vi "Process Outgoing Messages.vi"(0 "J1939 Cluster":T10, 1 "Connection Refs":T1, 5 "Timeouts":T9[](array[typedef]) {"Arb ID" format="%.0x"}, 7 "Data Ref":T7, 9 "Scale Ref":T8, 11 "error in":errorcluster, 12 "timeout in ms (-1)":i32=10) -> (4 "J1939 Cluster Out":T10, 13 "Message Errors":errorcluster, 15 "error out":errorcluster)   [LabVIEW 2015, in "J1939 Addon Engine.lvlib"]
uses:
  J1939 Addon Engine.lvlib
  Types/Setup Information Cluster.ctl
  <vilib>/xnet/xnet.llb/XNET Frame CAN.ctl
  <vilib>/xnet/xnet.llb/XNET Frame Type CAN.ctl
  Shared/J1939 Utilities/Types/CAN Outgoing Message Cluster.ctl
  J1939 Periodic Messages/SubVIs/Periodic Message Generator Cluster.ctl
  Types/Conversion Lookup Table Reference.ctl
  Types/Data Lookup Table Reference.ctl
  Types/Datatable Lookup DVR.ctl
  Types/TP List References.ctl
  Types/BAM Buffer Connections List_Ref.ctl
  Types/TP Buffer Connection Cluster.ctl
  Types/Connection Mode Generation Connection Ref.ctl
  Types/Connection Mode Generation Connection Cluster.ctl
  Types/BAM Generation Connections List_Ref.ctl
  Types/BAM Generation Connection Cluster.ctl
  Types/Address Table Reference.ctl
  Types/RQST Lookup Table Reference.ctl
  Shared/J1939 Utilities/Check Output Message Frame Type.vi
  J1939 Multi Packet Frames/BAM Generation.vi
  SubVIs/BAM Generation Connections List_Actions.vi
  SubVIs/BAM Generation Create New TP Connection.vi
  J1939 Multi Packet Frames/Connection Mode Generation.vi
  SubVIs/Connection Mode Generation Connections List_Actions.vi
  SubVIs/Connection Mode Generation Search for Connection (Local Message).vi
  SubVIs/Connection Mode Generation Create New TP Connection.vi
  Convert Signals to Frame by ID.vi
  Shared/J1939 Utilities/Common Conversions.vi
  Shared/J1939 Utilities/SubVIs/Convert CAN Arb ID to J1939 ID.vi
  Shared/J1939 Utilities/Common Messages.vi
  Shared/J1939 Utilities/SubVIs/TP.CM BAM.vi
  Shared/J1939 Utilities/SubVIs/TP.DT.vi
  Shared/J1939 Utilities/SubVIs/TP.CM RTS.vi
  Conversion Lookup Table Get Conversion Parameter.vi
  Data Lookup Table Get Signals (Range).vi
  Shared/J1939 Utilities/SubVIs/Convert J1939 ID to CAN Arb ID.vi
  SubVIs/Connection Mode Generation Connections List.vi
  SubVIs/BAM Generation Connections List.vi
  SubVIs/BAM Generation Search for Connection (Local Message).vi
  <vilib>/xnet/xnet.llb/XNET Convert.vi
  <vilib>/xnet/xnet.llb/XNET Convert (Signal to Frame CAN).vi
  Data Lookup Table.vi
  Conversion Lookup Table.vi
  Shared/J1939 Utilities/J1939 Utilities.lvlib
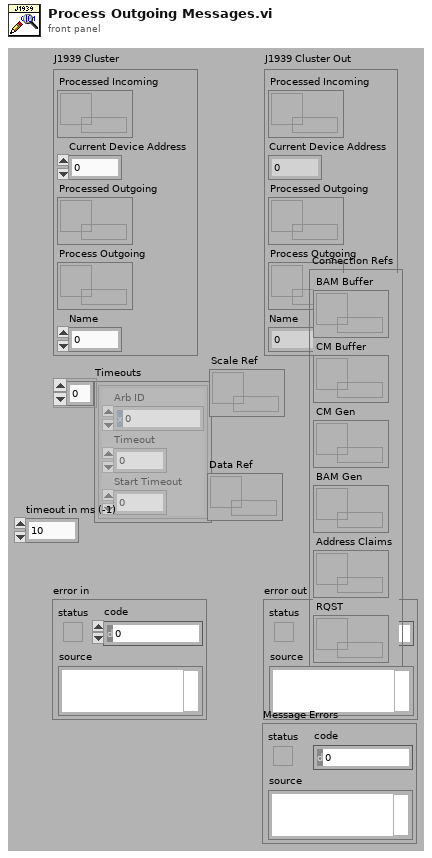
[diagram p1: front panel]
types:
  T1 = typedef "J1939 Addon Engine.lvlib/TP List References.ctl" = cluster{"BAM Buffer":T2, "CM Buffer":T2, "CM Gen":T3, "BAM Gen":T4, "Address Claims":T5, "RQST":T6}
  T2 = typedef "J1939 Addon Engine.lvlib/BAM Buffer Connections List_Ref.ctl" = refnum<data-value>
  T3 = typedef "J1939 Addon Engine.lvlib/Connection Mode Generation Connection Ref.ctl" = refnum<data-value>
  T4 = typedef "J1939 Addon Engine.lvlib/BAM Generation Connections List_Ref.ctl" = refnum<data-value>
  T5 = typedef "J1939 Addon Engine.lvlib/Address Table Reference.ctl" = refnum<data-value>
  T6 = typedef "J1939 Addon Engine.lvlib/RQST Lookup Table Reference.ctl" = refnum<data-value>
  T7 = typedef "J1939 Addon Engine.lvlib/Data Lookup Table Reference.ctl" = refnum<data-value>
  T8 = typedef "J1939 Addon Engine.lvlib/Conversion Lookup Table Reference.ctl" = refnum<data-value>
  T9 = typedef "J1939 Addon Engine.lvlib/Periodic Message Generator Cluster.ctl" = cluster{"Arb ID":u32, "Timeout":u32, "Start Timeout":u32}
  T10 = typedef "J1939 Addon Engine.lvlib/Setup Information Cluster.ctl" = cluster{"Processed Incoming":refnum<queue>, "Current Device Address":u8, "Processed Outgoing":refnum<queue>, "Process Outgoing":refnum<queue>, "Name":u64}
  T11 = typedef "J1939 Addon Shared.lvlib/J1939 Utilities.lvlib/CAN Outgoing Message Cluster.ctl" = cluster{"Identifier":u32, "Data":u8[]}
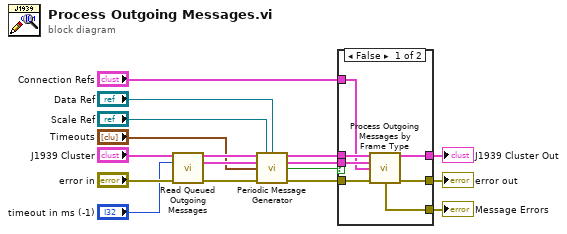
[diagram p0: block diagram]
diagram:
  n1 = call "Read Queued Outgoing Messages.vi"("J1939 Cluster"="J1939 Cluster", "timeout in ms (-1)"="timeout in ms (-1)", "error in"="error in") -> ("J1939 Cluster Out"=w11:T10, "Output Array"=w9:T11[], "error out"=w13:errorcluster)  [unwired: 1 in, 9 out]
  n2 = call "Periodic Message Generator.vi"("J1939 Cluster"=w11, "Scale Ref"="Scale Ref", "Data Ref"="Data Ref", "Output Array"=w9, "Timeouts"="Timeouts", "error in"=w13) -> ("J1939 Cluster Out"=w10:T10, "Output Array"=w8:T11[], "Empty?"=w7:bool, "error out"=w12:errorcluster)  [unwired: 6 out]
  n3 = case shown="False" w7 {
    tunnel: [w24 w25] -> w14
    tunnel: [w23 w26] -> w15
    tunnel: w10 -> [w22 w25]
    tunnel: w8 -> [w21 _]
    tunnel: w12 -> [w20 w26]
    tunnel: "Connection Refs" -> [w19 _]
    tunnel: [w18 _] -> w2
    frame False {
      n4 = call "Process Outgoing Messages by Frame Type.vi"("J1939 Cluster"=w22, "Output Array"=w21, "Connection Refs"=w19, "error in"=w20) -> ("J1939 Cluster"=w24:T10, "Message Errors"=w18:errorcluster, "System Error"=w23:errorcluster)  [unwired: 9 out]
    }
    frame True {
    }
  }
  "error out" <- w15
  "J1939 Cluster Out" <- w14
  "Message Errors" <- w2
